vi "Cannon Process.vi"(0 "error in":errorcluster) -> ()   [LabVIEW 2012]
uses:
  Cannon Global Data.vi
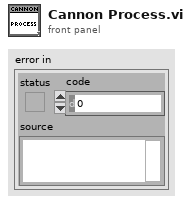
[diagram p1: front panel]
types:
  T1 = cluster{"Throttle":dbl, "RPM":dbl, "Motor VBus":dbl}
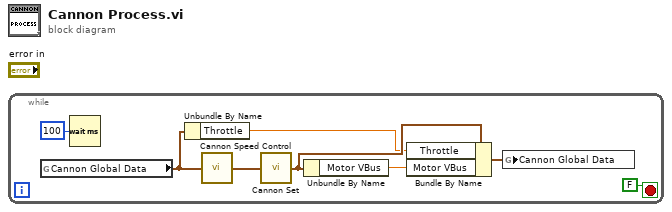
[diagram p0: block diagram]
diagram:
  n1 = while {
    stop <- FALSE stop-if-true
    n2 = global read "Cannon Global Data.vi" "Cannon Global Data"() -> (w2:T1)
    n3 = Wait (ms)(milliseconds to wait=100) -> ()  [unwired: 1 out]
    n4 = Unbundle By Name(w2) -> ("Throttle"=w4:dbl)
    n5 = call "Cannon Speed Control.vi"("Cannon Global Data In"=w2) -> ("Cannon Global Data Out"=w6:T1)
    n6 = call "Cannon Set.vi"("Cannon Global Data In"=w6) -> ("Cannon Global Data Out"=w5:T1)
    n7 = Unbundle By Name(w5) -> ("Motor VBus"=w1:dbl)
    n8 = Bundle By Name(cluster=w5, "Throttle"=w4, "Motor VBus"=w1) -> (w3:T1)
    n9 = global write "Cannon Global Data.vi" "Cannon Global Data"(w3) -> ()
  }
